vi "cmc-Series-While-Loop.vi"() -> ()   [LabVIEW 2010]
uses:
  <vilib>/gmath/NI_Gmath.lvlib
panel:
  out "Current Iteration":u8
  in  "Stop":bool
  in  "Delay Time (s)":dbl=1.0 min=0.0
  out "\"Canned Solution\"":dbl format="%#_18g"
  out "i-th term":dbl format="%#_18g"
  out "Partial Sum":dbl format="%#_18g"
  out "Total Summation":dbl format="%#_18g"
  in  "Number of Iterations\nRequested":u8
  in  "Theta(radians)":dbl
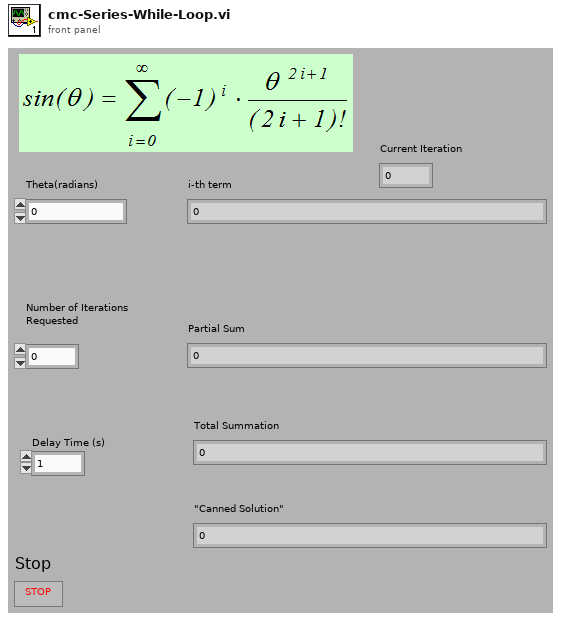
[diagram p1: front panel]
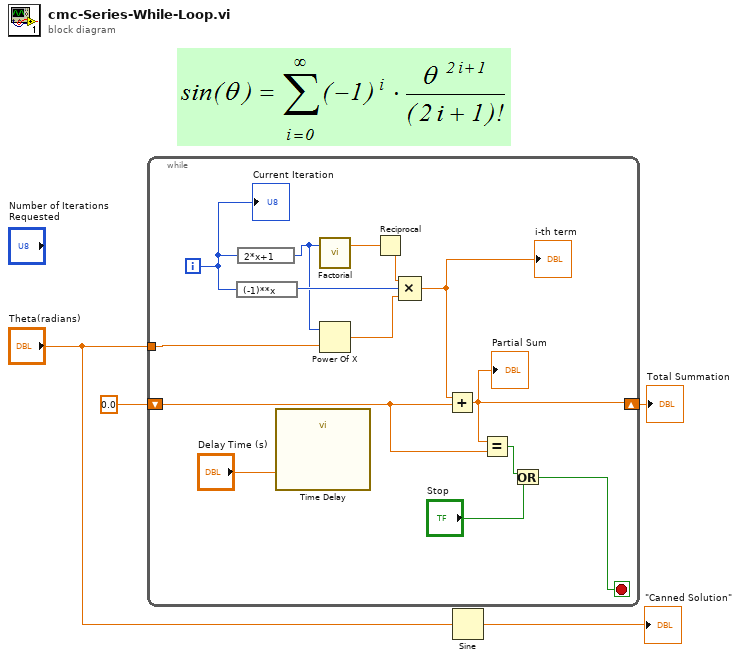
[diagram p0: block diagram]
diagram:
  n1 = while {
    tunnel: "Theta(radians)" -> [w13]
    shift-right: [w10] -> w3
    shift-left: 0.0 -> [w9]
    i -> [w5]
    stop <- w6 stop-if-true
    n2 = expression code="(-1)**x"(w5) -> (w17:i32)
    n3 = expression code="2*x+1"(w5) -> (w14:i32)
    n4 = call "Time Delay"("Delay Time (s)"="Delay Time (s)") -> ()  [unwired: 10 in, 1 out]
    n5 = call <vilib>:"Factorial.vi"("n"=w14) -> ("n!"=w15:dbl)  [unwired: 2 in]
    n6 = Power Of X(1:w13, 2:w14) -> (0:w16:dbl)
    n7 = Reciprocal(x=w15) -> (1/x=w18:dbl)
    n8 = Compound Arithmetic op=MULTIPLY(w18, w17, w16) -> (w12:dbl)
    "i-th term" <- w12
    n9 = Add(x=w12, y=w9) -> (x+y=w10:dbl)
    "Partial Sum" <- w10
    n10 = Equal?(x=w10, y=w9) -> (x = y?=w7:bool)
    n11 = Or(x=w7, y="Stop") -> (x .or. y?=w6:bool)
    "Current Iteration" <- w5
  }
  "Total Summation" <- w3
  n12 = Sine(x="Theta(radians)") -> (sin(x)=→"\"Canned Solution\"":dbl)
